vi "DIDPID XNET Conversion Global Properties.vi"(11 "DID/PID Selector":T1) -> (2 "Identifier":u32, 3 "signal name":string)   [LabVIEW 2015, in "Diagnostics Addon Engine.lvlib"]
uses:
  Diagnostics Addon Engine.lvlib
  Shared/Types/MessageType Selector.ctl
  Shared/Diagnostics Addon Shared.lvlib
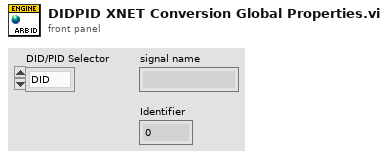
[diagram p1: front panel]
types:
  T1 = typedef "Diagnostics Addon Shared.lvlib/MessageType Selector.ctl" = enum16{"DID", "PID", "CPID", "Write Memory", "Read Memory", "DTC Control", "IO Cmd", "IO Resp", "Routine Start Cmd", "Routine Start Resp", "Routine Status Cmd", "Routine Status Resp", "Routine Stop Cmd", "Routine Stop Resp"}
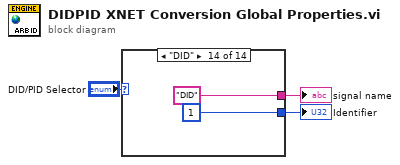
[diagram p0: block diagram]
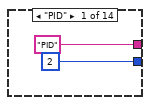
[diagram p2: hidden frame]
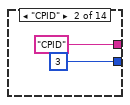
[diagram p3: hidden frame]
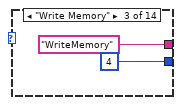
[diagram p4: hidden frame]
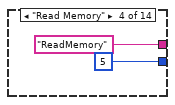
[diagram p5: hidden frame]
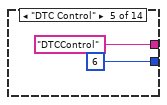
[diagram p6: hidden frame]
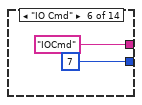
[diagram p7: hidden frame]
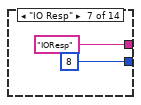
[diagram p8: hidden frame]
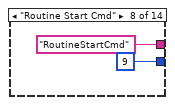
[diagram p9: hidden frame]
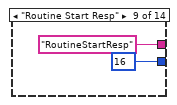
[diagram p10: hidden frame]
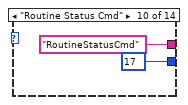
[diagram p11: hidden frame]
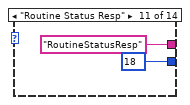
[diagram p12: hidden frame]
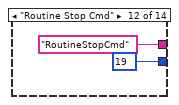
[diagram p13: hidden frame]
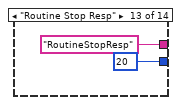
[diagram p14: hidden frame]
diagram:
  n1 = case shown="\"DID\"" "DID/PID Selector" {
    tunnel: ["PID" ("signal name") "CPID" ("signal name") "WriteMemory" ("signal name") "ReadMemory" ("signal name") "DTCControl" ("signal name") "IOCmd" ("signal name") "IOResp" ("signal name") "RoutineStartCmd" ("signal name") "RoutineStartResp" ("signal name") "RoutineStatusCmd" ("signal name") "RoutineStatusResp" ("signal name") "RoutineStopCmd" ("signal name") "RoutineStopResp" ("signal name") "DID" ("signal name")] -> w2
    tunnel: [u32 2 ("Identifier") u32 3 ("Identifier") u32 4 ("Identifier") u32 5 ("Identifier") u32 6 ("Identifier") u32 7 ("Identifier") u32 8 ("Identifier") u32 9 ("Identifier") u32 16 ("Identifier") u32 17 ("Identifier") u32 18 ("Identifier") u32 19 ("Identifier") u32 20 ("Identifier") u32 1 ("Identifier")] -> w1
    frame "PID" {
    }
    frame "CPID" {
    }
    frame "Write Memory" {
    }
    frame "Read Memory" {
    }
    frame "DTC Control" {
    }
    frame "IO Cmd" {
    }
    frame "IO Resp" {
    }
    frame "Routine Start Cmd" {
    }
    frame "Routine Start Resp" {
    }
    frame "Routine Status Cmd" {
    }
    frame "Routine Status Resp" {
    }
    frame "Routine Stop Cmd" {
    }
    frame "Routine Stop Resp" {
    }
    frame "DID" {
    }
  }
  "signal name" <- w2
  "Identifier" <- w1
